vi "Setup DO.vi"(0 "reference in":refnum<class "DO.lvclass">, 2 "Module Names (NI-MAX Alias)":string[](array[string])=["DO-Sink-32CH-1", "DO-Sink-32CH-2"], 3 "DAQ Port Number":u32, 4 "Number of Channels Per Module":u32[](array[numeric])=[32, 32], 5 "error in (no error)":errorcluster) -> (14 "reference out":refnum<class "DO.lvclass">, 16 "DO Task":refnum<k21>, 17 "Number of DO Modules":i32, 18 "Number of Total DO Channels":i32, 19 "error out":errorcluster)   [LabVIEW 2017, in "DO.lvclass"]
uses:
  DO.lvclass
  <vilib>/DAQmx/create/channels.llb/DAQmx Create Channel (DO-Digital Output).vi
  <resource>/objmgr/daqmx.rc
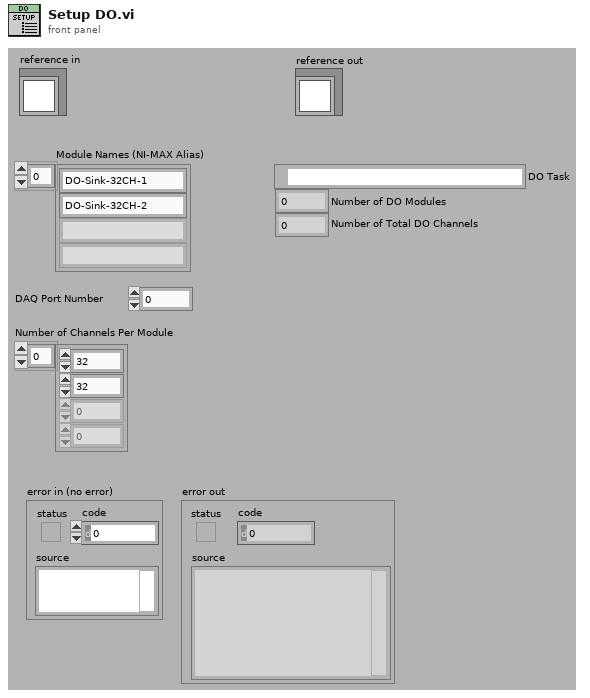
[diagram p1: front panel]
types:
  T1 = typedef "DO.lvclass/ObjectAttributes.ctl" = cluster{"DO Task":refnum<k21>, "DO Module Names (NI-Max Name)":string[], "Number of Channels Per DO Module":i32[], "DO Status":bool[], "Number of DO Modules":u32, "DO Status to Set":bool[], "DO On/Off Status":bool, "DO VI Reference":refnum<vi>, "Number of Total DO Channels":u32}
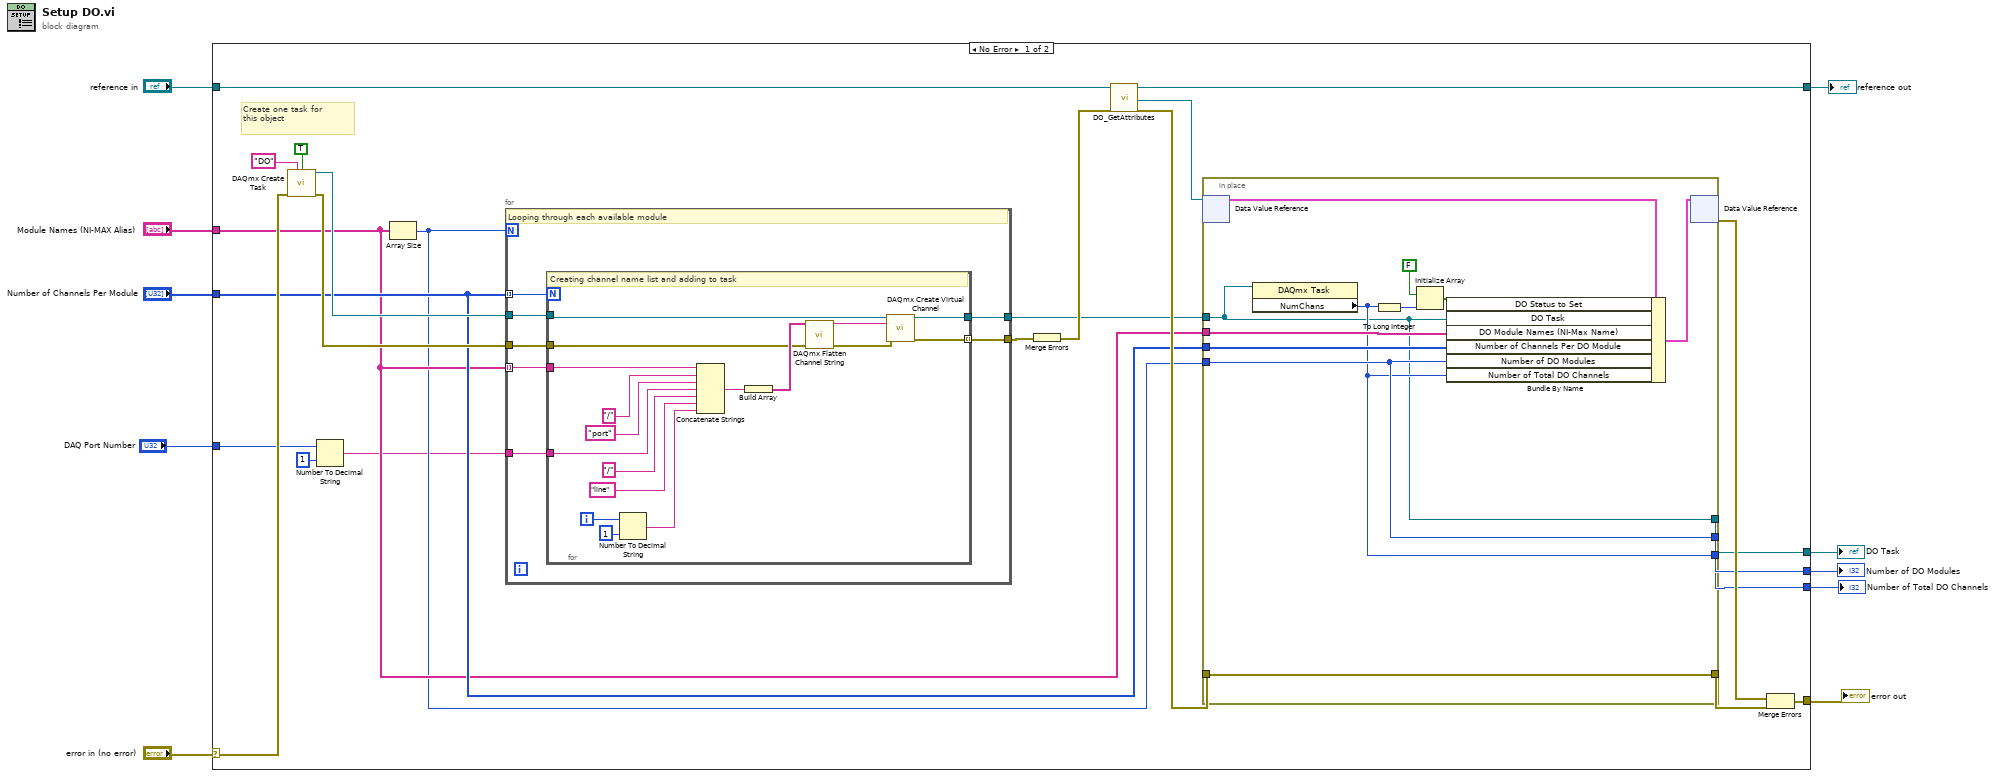
[diagram p0: block diagram]
diagram:
  n1 = case shown="No Error" "error in (no error)" {
    selector: "error in (no error)" -> [w25 w71]
    tunnel: [w31 w71] -> w9
    tunnel: [w32 w70] -> w7
    tunnel: "reference in" -> [w34 w70]
    tunnel: "Module Names (NI-MAX Alias)" -> [w19 _]
    tunnel: "Number of Channels Per Module" -> [w20 _]
    tunnel: [w17 _] -> w4
    tunnel: [w16 _] -> w3
    tunnel: [w15 _] -> w2
    tunnel: "DAQ Port Number" -> [w12 _]
    frame No Error {
      # "Create one task for \nthis object"
      n2 = call <vilib>:"DAQmx Create Task.vi"("new task name"="DO", "auto cleanup"=TRUE, "error in"=w25) -> ("task out"=w21:refnum<k21>, "error out"=w27:errorcluster)  [unwired: 11 in]
      n3 = Number To Decimal String(number=w12, width (-)=i16 1) -> (decimal integer string=w11:string)
      n4 = Array Size(array=w19) -> (size(s)=w18:i32)
      n5 = for {
        N: w18 -> [_]
        tunnel: w27 -> [w41]
        tunnel: [w40] -> w24
        tunnel: [w39] -> w22
        tunnel: w21 -> [w38]
        tunnel: w20 -> [w37] mode=indexing
        tunnel: w19 -> [w36] mode=indexing
        tunnel: w11 -> [w35]
        # "Looping through each available module"
        n6 = for {
          N: w37 -> [_]
          tunnel: w38 -> [w54]
          tunnel: [w53] -> w39
          tunnel: w41 -> [w49]
          tunnel: [w48] -> w40 mode=indexing
          tunnel: w36 -> [w47]
          tunnel: w35 -> [w42]
          i -> [w46]
          # "Creating channel name list and adding to task"
          n7 = Number To Decimal String(number=w46, width (-)=i16 1) -> (decimal integer string=w43:string)
          n8 = Concatenate Strings(w47, "/", "port", w42, "/", "line", w43) -> (w52:string)
          n9 = Build Array(w52) -> (w51:string[])
          n10 = call <vilib>:"DAQmx Flatten Channel String.vi"("names in"=w51, "error in"=w49) -> ("names out"=w55:string, "error out"=w56:errorcluster)  [unwired: 12 in]
          n11 = call-poly <vilib>:"DAQmx Create Virtual Channel.vi"("task in"=w54, "lines"=w55, "error in"=w56) -> ("task out"=w53:refnum<k21>, "error out"=w48:errorcluster)  [unwired: 11 in]
        }
      }
      n12 = Merge Errors(w24) -> (w23:errorcluster)
      n13 = call "DO_GetAttributes.vi"("reference in"=w34, "error in (no error)"=w23) -> ("reference out"=w32:refnum<class "DO.lvclass">, "DataRef"=w30:refnum<data-value>, "error out"=w29:errorcluster)  [unwired: 14 in, 1 out]
      n14 = in-place {
        in-place-border: w29 -> [w67]
        in-place-border: [w67] -> w28
        in-place-border: w22 -> [w59]
        in-place-border: w20 -> [w66]
        in-place-border: w19 -> [w65]
        in-place-border: w18 -> [w61]
        in-place-border: [w61] -> w17
        in-place-border: [w60] -> w16
        in-place-border: [w59] -> w15
        n15 = in-place-dvr #1(w30) -> (w68:T1)  [unwired: 1 out]
        n16 = property class="DAQmx Task"(reference=w59) -> ("NumChans"=w60:u32)  [unwired: 1 in, 2 out]
        n17 = To Long Integer(number=w60) -> (32bit integer=w62:i32)
        n18 = Initialize Array(FALSE, w62) -> (w64:bool[])
        n19 = Bundle By Name(cluster=w68, "DO Status to Set"=w64, "DO Task"=w59, "DO Module Names (NI-Max Name)"=w65, "Number of Channels Per DO Module"=w66, "Number of DO Modules"=w61, "Number of Total DO Channels"=w60) -> (w69:T1)
        n20 = in-place-dvr #1(w69) -> (w33:errorcluster)  [unwired: 1 out]
      }
      n21 = Merge Errors(w33, w28) -> (w31:errorcluster)
    }
    frame Error {
    }
  }
  "error out" <- w9
  "reference out" <- w7
  "Number of DO Modules" <- w4
  "Number of Total DO Channels" <- w3
  "DO Task" <- w2
